vi "get desired keys.vi"(8 "error in":errorcluster, 11 "LED configuration in":refnum<class "LED configuration.lvclass">) -> (0 "error out":errorcluster, 2 "desired keys":string[](array[string]), 3 "LED configuration out":refnum<class "LED configuration.lvclass">)   [LabVIEW 2013, in "LED configuration.lvclass"]
uses:
  LED configuration.lvclass
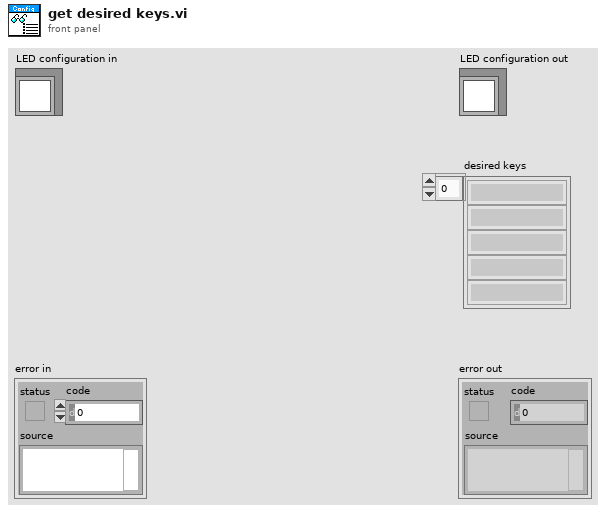
[diagram p1: front panel]
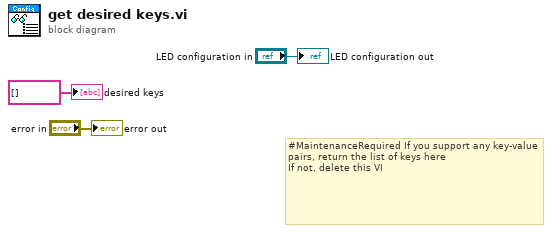
[diagram p0: block diagram]
diagram:
  # "#MaintenanceRequired If you support any key-value pairs, return the list of keys here\nIf not, delete this VI"
  "error out" <- "error in"
  "LED configuration out" <- "LED configuration in"
  "desired keys" <- string[] [] ("desired keys")
